vi "-8240 Invalid Instrument Identifier--error.vi"(8 "error in":errorcluster, 11 "Instrument Identifier":string) -> (0 "error out":errorcluster)   [LabVIEW 2020, in "Interactor.lvlib" / "Interactor.lvclass"]
uses:
  Interactor.lvclass
  Common-LabVIEW-Helpers/Source/Error Helpers.lvlib
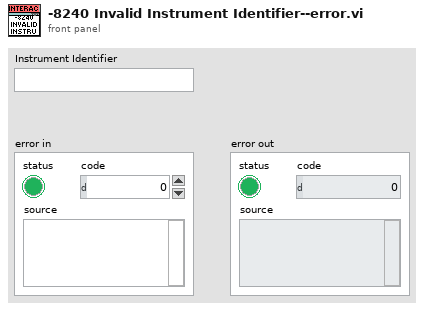
[diagram p1: front panel]
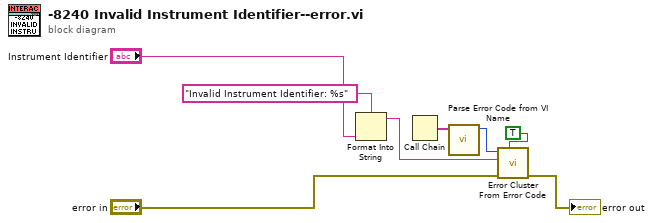
[diagram p0: block diagram]
diagram:
  n1 = Format Into String(format string="Invalid Instrument Identifier: %s" ("source"), "Instrument Identifier") -> (resulting string=w3:string)  [unwired: 2 in, 1 out]
  n2 = Call Chain() -> (call chain=w5:string[])
  n3 = call "Parse Error Code from VI Name.vi"("Call Chain"=w5) -> ("Error Code"=w4:i32)  [unwired: 10 in]
  n4 = call <vilib>:"Error Cluster From Error Code.vi"("show call chain? (False)"=TRUE, "error in (no error)"="error in", "error message (\"\")"=w3, "error code (0)"=w4) -> ("error out"=→"error out":errorcluster)  [unwired: 5 in]
